vi "Test App Adding Second Process and Starting App Again.vi"(8 "error in (no error)":errorcluster, 11 "Application Test In":refnum<class "Application Test.lvclass">) -> (0 "error out":errorcluster, 3 "Application Test Out":refnum<class "Application Test.lvclass">)   [LabVIEW 2020, in "Application Test.lvclass"]
uses:
  Application Test.lvclass
  C:/Program Files (x86)/National Instruments/LabVIEW 2020/vi.lib/Asteme/LUnit/Test Case.lvclass
  Mock Process/Mock Process.lvclass
  C:/Users/anton/Documents/GitHub/Triarc-Framework/source/Framework/Process/Process.lvclass
  Framework/Error Handler Interface/Error Handler Interface.lvclass
  Framework/Process/Process.lvclass/Process.ctl
  Framework/Application/Application.lvclass/Application.ctl
  <vilib>/Asteme/LUnit/Test Case.lvclass/Test Case.ctl
  <vilib>/Asteme/LUnit/LUnit Assertion Result.lvclass/LUnit Assertion Result.ctl
  Framework/Process/Public/Get Lifecycle State.vi
  Framework/Process/Protected/Messaging/Enqueue Message.vi
  <vilib>/Utility/error.llb/Clear Errors.vi
  Framework/Process/Protected/SubVIs/Set Context.vi
  Framework/Application/Private/Add Process to Map.vi
  Framework/Process/Private/SubVIs/Wait for finish.vi
  Framework/Process/Private/SubVIs/Set Lifecycle State.vi
  <vilib>/Asteme/LUnit/Palette/Fail.vi
  <vilib>/Asteme/LUnit/Palette/Pass.vi
  <vilib>/Asteme/LUnit/Set Assertion Type.vi
  <vilib>/AdvancedString/1D String Array to Delimited String.vi
  <vilib>/Asteme/LUnit/Add test result.vi
  <vilib>/Asteme/LUnit/LUnit Write Passed.vi
  <vilib>/Asteme/LUnit/LUnit Get Test Case.vi
  <vilib>/Asteme/LUnit/LUnit Write Message.vi
  <vilib>/Asteme/LUnit/LUnit Write Description.vi
  <vilib>/Asteme/LUnit/LUnit Write Assertion Type.vi
  <vilib>/Asteme/LUnit/Read Test Case Name.vi
  Framework/Application/Application.lvclass
  <vilib>/Utility/error.llb/Error Cluster From Error Code.vi
  <vilib>/Asteme/LUnit/Assertion Result/LUnit Get Test Name.vi
  Framework/Process/Process.lvclass
  <vilib>/Asteme/LUnit/LUnit Assertion Result.lvclass
  <vilib>/Asteme/LUnit/Test Case.lvclass
panel:
  out "Messages 2":string[](array[string])
  out "Messages":string[](array[string])
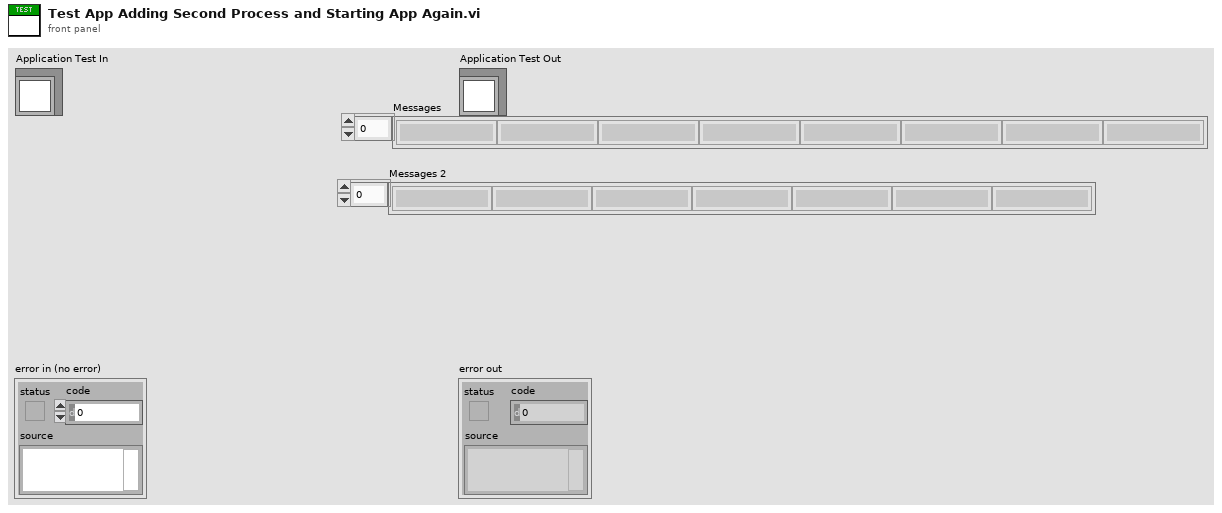
[diagram p1: front panel]
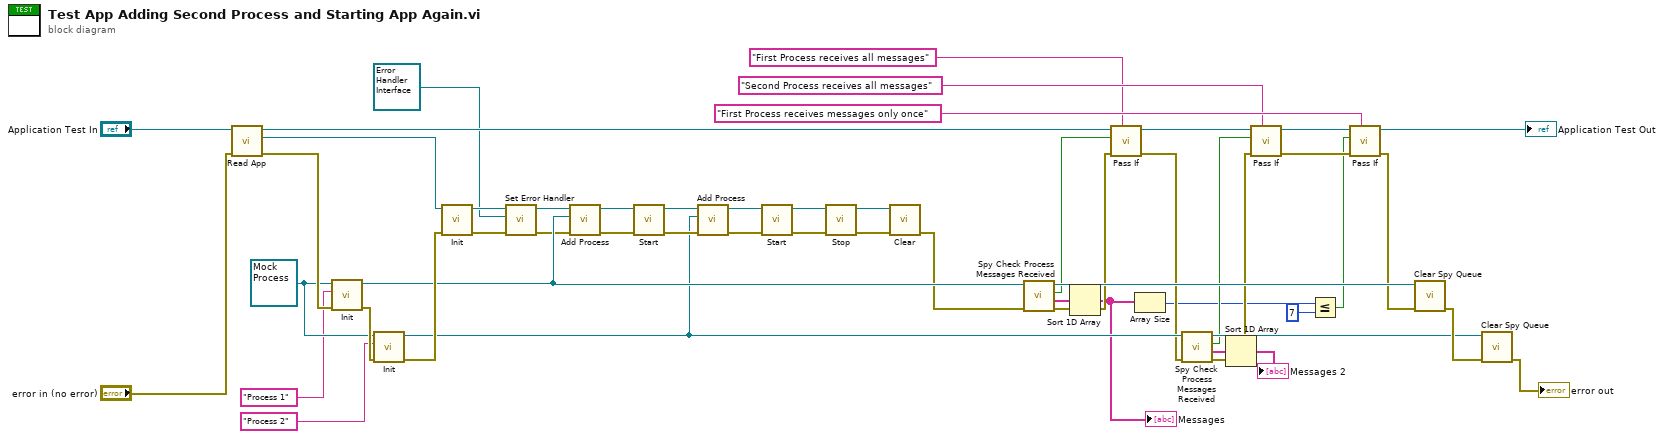
[diagram p0: block diagram]
diagram:
  w34 = refnum<class "Mock Process.lvclass"> refnum ("Mock Classes.lvlib:Mock Process.lvclass")
  n1 = call "Read App.vi"("error in (no error)"="error in (no error)", "Application Test In"="Application Test In") -> ("error out"=w37:errorcluster, "App out"=w38:refnum<class "Application.lvclass">, "Application Test Out"=w51:refnum<class "Application Test.lvclass">)  [unwired: 7 in]
  n2 = call-dynamic "Init.vi"("error in (no error)"=w37, "Name"="Process 1", "Mock Process In"=w34) -> ("error out"=w46:errorcluster, "Mock Process Out"=w42:refnum<class "Mock Process.lvclass">)  [unwired: 7 in]
  n3 = call-dynamic "Init.vi"("error in (no error)"=w46, "Name"="Process 2", "Mock Process In"=w34) -> ("error out"=w45:errorcluster, "Mock Process Out"=w28:refnum<class "Mock Process.lvclass">)  [unwired: 7 in]
  n4 = call-dynamic "Init.vi"("error in (no error)"=w45, "Process In"=w38) -> ("error out"=w8:errorcluster, "Process Out"=w49:refnum<class "Application.lvclass">)  [unwired: 8 in]
  n5 = call "Set Error Handler.vi"("error in (no error)"=w8, "Error Handler"=refnum<class "Error Handler Interface.lvclass"> refnum, "Process In"=w49) -> ("error out"=w7:errorcluster, "Process Out"=w9:refnum<class "Application.lvclass">)  [unwired: 7 in]
  n6 = call "Add Process.vi"("error in (no error)"=w7, "Process"=w42, "Rig In"=w9) -> ("error out"=w30:errorcluster, "Rig Out"=w33:refnum<class "Application.lvclass">)  [unwired: 7 in]
  n7 = call "Start.vi"("error in (no error)"=w30, "Process In"=w33) -> ("error out"=w31:errorcluster, "Process Out"=w32:refnum<class "Application.lvclass">)  [unwired: 8 in]
  n8 = call "Add Process.vi"("error in (no error)"=w31, "Process"=w28, "Rig In"=w32) -> ("error out"=w39:errorcluster, "Rig Out"=w40:refnum<class "Application.lvclass">)  [unwired: 7 in]
  n9 = call "Start.vi"("error in (no error)"=w39, "Process In"=w40) -> ("error out"=w35:errorcluster, "Process Out"=w36:refnum<class "Application.lvclass">)  [unwired: 8 in]
  n10 = call "Stop.vi"("error in (no error)"=w35, "Process In"=w36) -> ("error out"=w47:errorcluster, "Process Out"=w48:refnum<class "Application.lvclass">)  [unwired: 7 in, 1 out]
  n11 = call-dynamic "Clear.vi"("error in (no error)"=w47, "Application In"=w48) -> ("error out"=w41:errorcluster)  [unwired: 8 in, 1 out]
  n12 = call "Spy Check Process Messages Received.vi"("error in (no error)"=w41, "Mock Process In"=w42) -> ("error out"=w24:errorcluster, "Messages"=w15:string[], "Messages received?"=w22:bool, "Mock Process Out"=w29:refnum<class "Mock Process.lvclass">)  [unwired: 6 in]
  n13 = Sort 1D Array(array=w15) -> (sorted array=w4:string[])
  "Messages" <- w4
  n14 = call <vilib>:"Pass If.vi"("Description"="First Process receives all messages", "error in (no error)"=w24, "Pass?"=w22, "Test Case In"=w51) -> ("error out"=w23:errorcluster, "Test Case Out"=w26:refnum<class "Application Test.lvclass">)  [unwired: 6 in]
  n15 = Array Size(array=w4) -> (size(s)=w3:i32)
  n16 = call "Spy Check Process Messages Received.vi"("error in (no error)"=w23, "Mock Process In"=w28) -> ("error out"=w19:errorcluster, "Messages"=w18:string[], "Messages received?"=w20:bool, "Mock Process Out"=w27:refnum<class "Mock Process.lvclass">)  [unwired: 6 in]
  n17 = Sort 1D Array(array=w18) -> (sorted array=→"Messages 2":string[])
  n18 = call <vilib>:"Pass If.vi"("Description"="Second Process receives all messages", "error in (no error)"=w19, "Pass?"=w20, "Test Case In"=w26) -> ("error out"=w17:errorcluster, "Test Case Out"=w25:refnum<class "Application Test.lvclass">)  [unwired: 6 in]
  n19 = Less Or Equal?(x=w3, y=7) -> (x <= y?=w1:bool)
  n20 = call <vilib>:"Pass If.vi"("Description"="First Process receives messages only once", "error in (no error)"=w17, "Pass?"=w1, "Test Case In"=w25) -> ("error out"=w16:errorcluster, "Test Case Out"=→"Application Test Out":refnum<class "Application Test.lvclass">)  [unwired: 6 in]
  n21 = call-dynamic "Clear Spy Queue.vi"("error in (no error)"=w16, "Mock Process In"=w29) -> ("error out"=w44:errorcluster)  [unwired: 8 in, 1 out]
  n22 = call-dynamic "Clear Spy Queue.vi"("error in (no error)"=w44, "Mock Process In"=w27) -> ("error out"=→"error out":errorcluster)  [unwired: 8 in, 1 out]
